vi "Magnetic Sweep 1.9.vi"() -> ()   [LabVIEW 2011]
panel:
  out "Current time":timestamp format="%<%I:%M:%S %p\n%x>T"
  out "error out":errorcluster
  in  "error in (no error) 2":errorcluster
  out "x .and. y?":bool
  in  "Initial Temperature":dbl
  out "Heater":bool
  out "Persistent switch ready":bool
  out "error out 6":errorcluster
  in  "Temperature\nlower limite":dbl
  out "Ramping rate command":string
  out "Target field command":string
  out "String":string="Persistent switch is not on"
  in  "Set parameter":bool
  out "status":string
  out "PID command":string
  out "setpoint command":string
  out "setpoint":dbl
  in  "stop":bool
  out "error out 3":errorcluster
  out "error out 2":errorcluster
  in  "Contour plot (ramp down)":path
  in  "Raw data (ramp down)":path
  out "Elapsed Time (s)":dbl format="%#_1g"
  out "Iteration":i32
  out "Zero field reached":bool
  out "Target field reached":bool
  in  "Temperature\nupper limite":dbl
  in  "Temperature\nramping step":dbl
  in  "Heater range":i16(ring) items=["High", "Medium", "Low"]
  in  "D gain":dbl
  in  "I gain":dbl
  in  "P gain":dbl
  in  "Contour plot (ramp up)":path
  in  "Timer":bool caption="Reset"
  in  "date format":enum16{"short", "long", "abbreviated"}(ring)
  in  "Save":bool
  in  "Raw data (ramp  up)":path
  out "Current Resistance":string
  out "Current Temperature":string
  out "Current Field":string
  out "Status":string
  in  "Field Sweep":bool
  in  "Magnetic field\nRamp rate":dbl
  in  "Traget Field":dbl
  out "Init Response":string
  in  "error in (no error)":errorcluster
  in  "IP Address":string
  in  "Update":bool
  in  "P Switch":bool
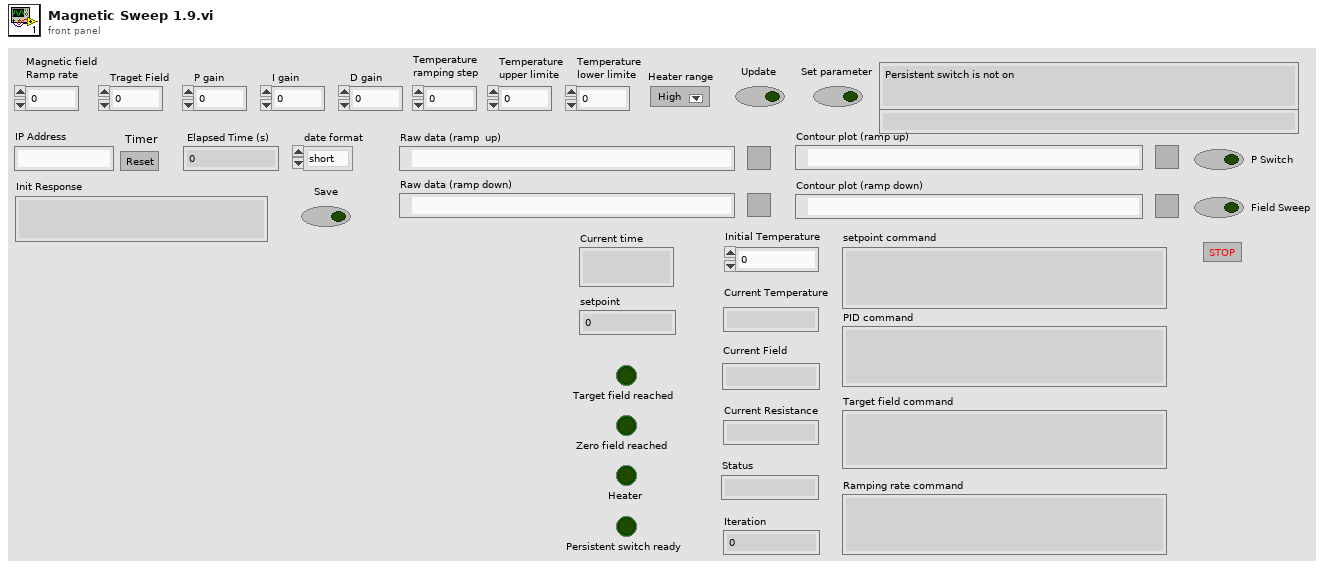
[diagram p1: front panel]
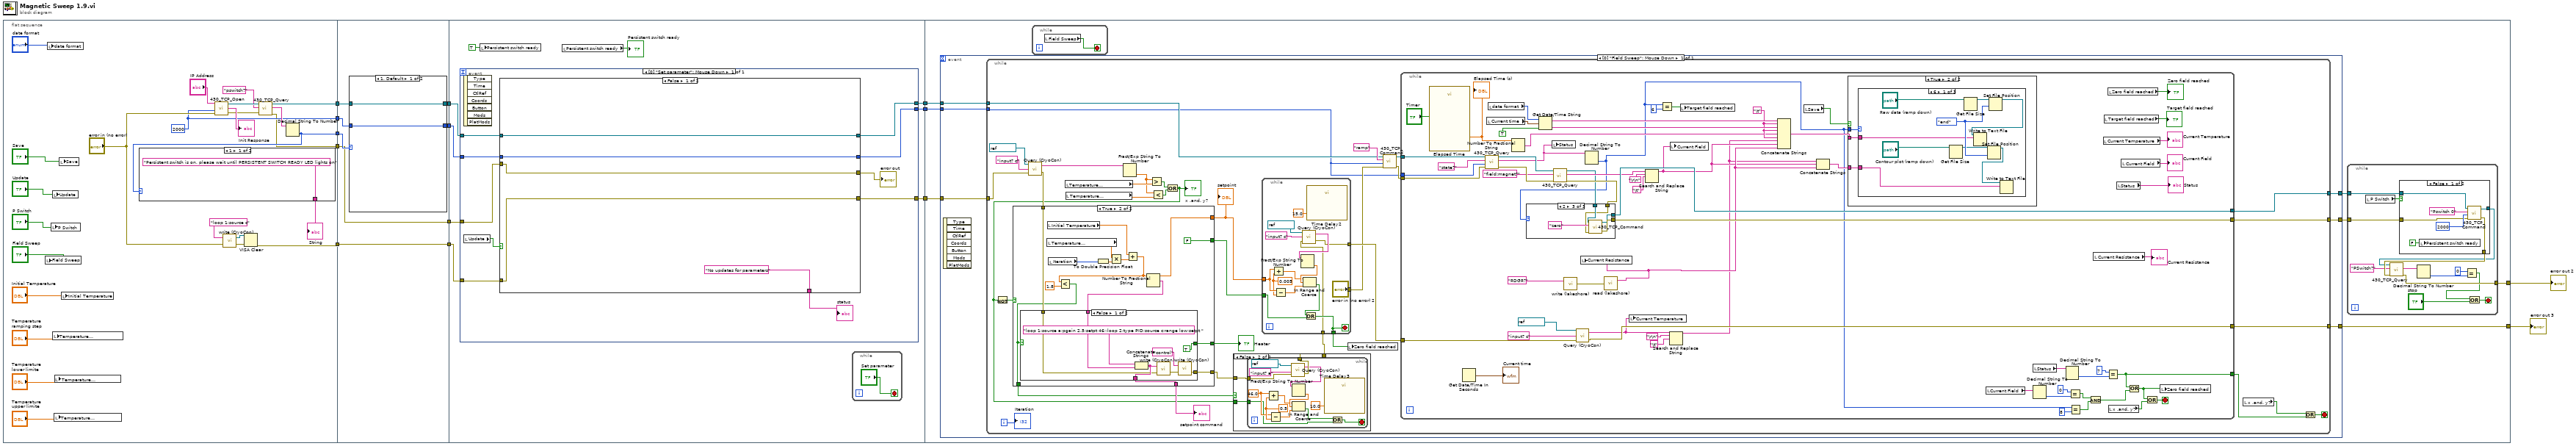
[diagram p0: block diagram]
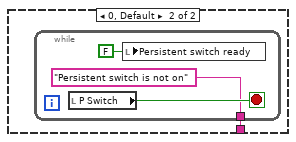
[diagram p2: hidden frame]
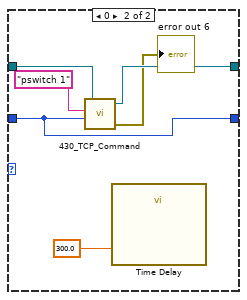
[diagram p3: hidden frame]
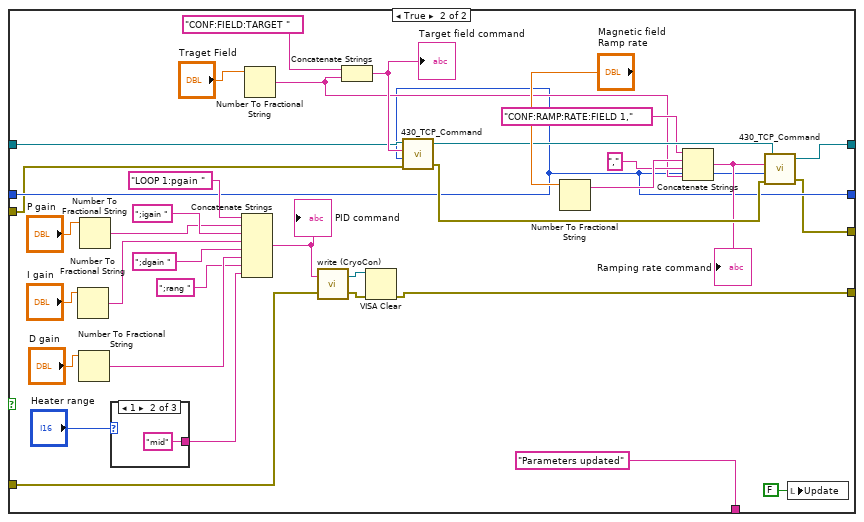
[diagram p4: hidden frame]
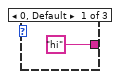
[diagram p5: hidden frame]
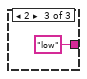
[diagram p6: hidden frame]
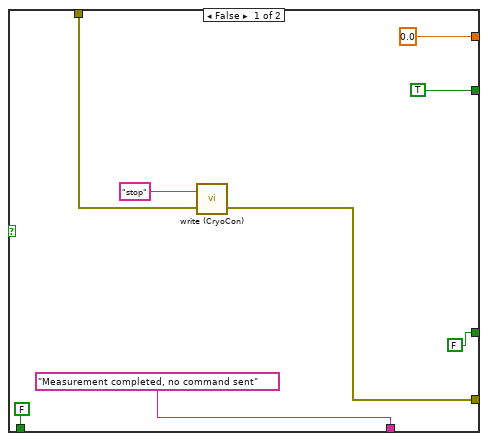
[diagram p9: hidden frame]
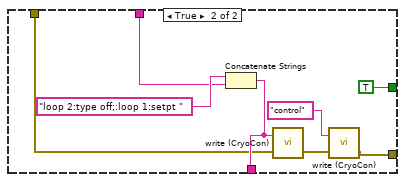
[diagram p10: hidden frame]
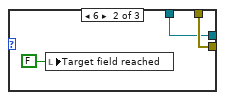
[diagram p12: hidden frame]
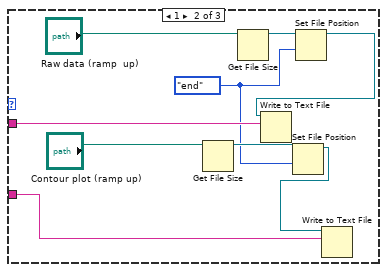
[diagram p14: hidden frame]
diagram:
  n1 = flat-sequence {
    tunnel: [w19] -> w11
    tunnel: [w21] -> w9
    tunnel: [w23] -> w7
    tunnel: [w18] -> w5
    tunnel: [w15] -> w1
    tunnel: w11 -> [w50]
    tunnel: [w48] -> w10
    tunnel: w9 -> [w49]
    tunnel: [w46] -> w8
    tunnel: w7 -> [w51]
    tunnel: [w51] -> w6
    tunnel: w5 -> [w47]
    tunnel: [w45] -> w2
    tunnel: w1 -> [w45]
    tunnel: w10 -> [w61]
    tunnel: w8 -> [w68]
    tunnel: w6 -> [w67]
    tunnel: [w66] -> w14
    tunnel: [w65] -> w13
    tunnel: [w64] -> w12
    tunnel: w2 -> [w60]
    tunnel: w14 -> [w129]
    tunnel: w13 -> [w126]
    tunnel: w12 -> [w125]
    tunnel: [w124] -> w4
    tunnel: [w123] -> w3
    frame #0 {
      w21 = 2000 ("Timeout")
      n2 = local write "Field Sweep"("Field Sweep") -> ()
      n3 = local write "date format"("date format") -> ()
      n4 = local write "P Switch"("P Switch") -> ()
      n5 = local write "Update"("Update") -> ()
      n6 = local write "Temperature\nramping step"("Temperature\nramping step") -> ()
      n7 = local write "Temperature\nupper limite"("Temperature\nupper limite") -> ()
      n8 = local write "Temperature\nlower limite"("Temperature\nlower limite") -> ()
      n9 = local write "Save"("Save") -> ()
      n10 = local write "Initial Temperature"("Initial Temperature") -> ()
      n11 = call "430_TCP_Open.vi"("IP Address"="IP Address", "timeout ms (2000)"=w21, "error in (no error)"="error in (no error)") -> ("connection ID"=w29:refnum<k5>, "Init Response"=→"Init Response":string, "error out"=w28:errorcluster)  [unwired: 3 in]
      n12 = call "write (CryoCon).vi"("error in (no error)"="error in (no error)", "write buffer"="loop 1:source c") -> ("error out"=w25:errorcluster, "VISA resource name out"=w24:refnum<visa-resource-name>)
      n13 = VISA Clear(VISA resource name=w24, error in (no error)=w25) -> (error out=w23:errorcluster)  [unwired: 1 out]
      n14 = call "430_TCP_Query.vi"("error in (no error)"=w28, "Command"="pswitch?", "connection ID"=w29) -> ("error out"=w15:errorcluster, "Response"=w26:string, "connection ID out"=w19:refnum<k5>)  [unwired: 4 in, 2 out]
      n15 = Decimal String To Number(string=w26) -> (number=w18:i32)  [unwired: 2 in, 1 out]
      n16 = case shown="1" w18 {
        tunnel: ["Persistent switch is on, please wait until PERSISTENT SWITCH READY LED lights on" w41] -> w22
        frame 1 {
        }
        frame 0, Default {
          n17 = while {
            tunnel: ["Persistent switch is not on"] -> w41
            stop <- w44 stop-if-true
            n18 = local read "P Switch"() -> (w44:bool)
            n19 = local write "Persistent switch ready"(FALSE ("Persistent switch ready")) -> ()
          }
        }
      }
      "String" <- w22
    }
    frame #1 {
      n20 = case shown="1, Default" w47 {
        tunnel: w50 -> [w53 w59]
        tunnel: w49 -> [w52 w54]
        tunnel: [w53 w58] -> w48
        tunnel: [w52 w54] -> w46
        frame 1, Default {
        }
        frame 0 {
          n21 = call "430_TCP_Command.vi"("Timeout"=w54, "Command"="pswitch 1", "connection ID"=w59) -> ("error out"=→"error out 6":errorcluster, "connection ID out"=w58:refnum<k5>)  [unwired: 1 in, 1 out]
          n22 = call "Time Delay"("Delay Time (s)"=300.0) -> ()  [unwired: 10 in, 1 out]
        }
      }
    }
    frame #2 {
      n23 = event shown="[0] \"Set parameter\": Mouse Down" {
        selector: _ -> [_]
        dyn-events: _ -> [_]
        timeout: _ -> [_]
        tunnel: w61 -> [w79]
        tunnel: w68 -> [w78]
        tunnel: w67 -> [w77]
        tunnel: [w76] -> w66
        tunnel: [w75] -> w65
        tunnel: [w74] -> w64
        tunnel: w60 -> [w71]
        event "Set parameter": Mouse Down {
          n24 = event-data() -> ()  [unwired: 1 in, 7 out]
          n25 = local read "Update"() -> (w72:bool)
          n26 = case shown="False" w72 {
            tunnel: w79 -> [w82 w117]
            tunnel: w78 -> [w83 w90]
            tunnel: w77 -> [w81 w96]
            tunnel: [w81 w86] -> w76
            tunnel: ["No updates for parameters" ("String") "Parameters updated" ("String")] -> w73
            tunnel: [w82 w91] -> w75
            tunnel: [w83 w90] -> w74
            tunnel: w71 -> [w80 w87]
            tunnel: [w80 w85] -> w70
            frame False {
            }
            frame True {
              n27 = Number To Fractional String(number="I gain") -> (F-format string=w100:string)  [unwired: 3 in]
              n28 = Number To Fractional String(number="D gain") -> (F-format string=w98:string)  [unwired: 3 in]
              n29 = Number To Fractional String(number="P gain") -> (F-format string=w101:string)  [unwired: 3 in]
              n30 = case shown="1" "Heater range" {
                tunnel: ["hi" "mid" "low"] -> w93
                frame 0, Default {
                }
                frame 1 {
                }
                frame 2 {
                }
              }
              n31 = Concatenate Strings("LOOP 1:pgain " ("write buffer"), w101, ";igain " ("string"), w100, ";dgain " ("string"), w98, ";rang " ("string"), w93) -> (w97:string)
              "PID command" <- w97
              n32 = Number To Fractional String(number="Traget Field") -> (F-format string=w107:string)  [unwired: 3 in]
              n33 = call "write (CryoCon).vi"("error in (no error)"=w96, "write buffer"=w97) -> ("error out"=w89:errorcluster, "VISA resource name out"=w88:refnum<visa-resource-name>)
              n34 = Concatenate Strings("CONF:FIELD:TARGET ", w107) -> (w118:string)
              "Target field command" <- w118
              n35 = VISA Clear(VISA resource name=w88, error in (no error)=w89) -> (error out=w86:errorcluster)  [unwired: 1 out]
              n36 = call "430_TCP_Command.vi"("error in (no error)"=w87, "Timeout"=w90, "Command"=w118, "connection ID"=w117) -> ("error out"=w116:errorcluster, "connection ID out"=w112:refnum<k5>)  [unwired: 1 out]
              n37 = Number To Fractional String(number="Magnetic field\nRamp rate") -> (F-format string=w110:string)  [unwired: 3 in]
              n38 = Concatenate Strings("CONF:RAMP:RATE:FIELD 1," ("string"), w110, "," ("string"), w107) -> (w113:string)
              "Ramping rate command" <- w113
              n39 = call "430_TCP_Command.vi"("error in (no error)"=w116, "Timeout"=w90, "Command"=w113, "connection ID"=w112) -> ("error out"=w85:errorcluster, "connection ID out"=w91:refnum<k5>)  [unwired: 1 out]
              n40 = local write "Update"(FALSE ("Update")) -> ()
            }
          }
          "status" <- w73
          "error out" <- w70
        }
      }
      n41 = local write "Persistent switch ready"(TRUE ("Persistent switch ready")) -> ()
      n42 = local read "Persistent switch ready"() -> (→"Persistent switch ready":bool)
      n43 = while {
        stop <- "Set parameter" stop-if-true
      }
    }
    frame #3 {
      n44 = event shown="[0] \"Field Sweep\": Mouse Down" {
        selector: _ -> [_]
        dyn-events: _ -> [_]
        timeout: _ -> [_]
        tunnel: w129 -> [w158]
        tunnel: [w157] -> w128
        tunnel: [w156] -> w127
        tunnel: w126 -> [w155]
        tunnel: w125 -> [w154]
        tunnel: [w153] -> w124
        event "Field Sweep": Mouse Down {
          n45 = event-data() -> ()  [unwired: 1 in, 7 out]
          n46 = while {
            tunnel: w158 -> [w175]
            tunnel: [w169] -> w157
            tunnel: [w188] -> w156
            tunnel: w155 -> [w187]
            tunnel: w154 -> [w159]
            tunnel: [w170] -> w153
            i -> [w191]
            stop <- w176 stop-if-true
            n47 = call "Query (CryoCon).vi"("error in (no error)"=w175, "write buffer"="input? c", "VISA resource name 2"=refnum<visa-resource-name> "COM3") -> ("error out"=w173:errorcluster, "read buffer"=w185:string)
            n48 = local read "Temperature\nupper limite"() -> (w189:dbl)
            n49 = local read "Temperature\nlower limite"() -> (w182:dbl)
            n50 = Fract/Exp String To Number(string=w185) -> (number=w183:dbl)  [unwired: 3 in, 1 out]
            n51 = Greater?(x=w183, y=w189) -> (0:w180:bool)
            n52 = Less?(x=w183, y=w182) -> (x < y?=w181:bool)
            n53 = Or(x=w180, y=w181) -> (x .or. y?=w160:bool)
            "x .and. y?" <- w160
            n54 = Not(x=w160) -> (.not. x?=w172:bool)
            n55 = case shown="True" w172 {
              tunnel: [w227 w242] -> w162
              tunnel: [0.0 w240] -> w192
              tunnel: ["Measurement completed, no command sent" w243] -> w171
              tunnel: [TRUE FALSE] -> w179
              tunnel: w173 -> [w229 w236]
              tunnel: [FALSE ("Heater") w235] -> w164
              tunnel: [FALSE w234] -> w163
              frame False {
                n56 = call "write (CryoCon).vi"("error in (no error)"=w229, "write buffer"="stop") -> ("error out"=w227:errorcluster)  [unwired: 1 out]
              }
              frame True {
                n57 = local read "Temperature\nramping step"() -> (w245:dbl)
                n58 = local read "Initial Temperature"() -> (w238:dbl)
                n59 = local read "Iteration"() -> (w237:i32)
                n60 = To Double Precision Float(number=w237) -> (double precision float=w244:dbl)
                n61 = Multiply(x=w245, y=w244) -> (x*y=w246:dbl)
                n62 = Add(x=w238, y=w246) -> (x+y=w240:dbl)
                n63 = Less?(x=w240, y=1.8) -> (x < y?=w234:bool)
                n64 = Number To Fractional String(number=w240) -> (F-format string=w247:string)  [unwired: 3 in]
                n65 = case shown="False" w234 {
                  tunnel: w247 -> [w254 w262]
                  tunnel: [w251 w261] -> w243
                  tunnel: [w253 w260] -> w242
                  tunnel: w236 -> [w248 w257]
                  tunnel: [TRUE ("Heater") TRUE ("Heater")] -> w235
                  frame False {
                    n66 = Concatenate Strings("loop 1:source a;pgain 2.5;setpt 46;:loop 2:type PID;source c;range low;setpt " ("write buffer"), w254) -> (w251:string)
                    n67 = call "write (CryoCon).vi"("error in (no error)"=w248, "write buffer"=w251) -> ("error out"=w250:errorcluster)  [unwired: 1 out]
                    n68 = call "write (CryoCon).vi"("error in (no error)"=w250, "write buffer"="control") -> ("error out"=w253:errorcluster)  [unwired: 1 out]
                  }
                  frame True {
                    n69 = Concatenate Strings("loop 2:type off;:loop 1:setpt " ("write buffer"), w262) -> (w261:string)
                    n70 = call "write (CryoCon).vi"("error in (no error)"=w257, "write buffer"=w261) -> ("error out"=w259:errorcluster)  [unwired: 1 out]
                    n71 = call "write (CryoCon).vi"("error in (no error)"=w259, "write buffer"="control") -> ("error out"=w260:errorcluster)  [unwired: 1 out]
                  }
                }
              }
            }
            "setpoint" <- w192
            "setpoint command" <- w171
            "Heater" <- w164
            n72 = case shown="False" w163 {
              tunnel: w162 -> [w193 w196]
              tunnel: [w193 w195] -> w161
              tunnel: w160 -> [_ w194]
              frame True {
              }
              frame False {
                n73 = while {
                  tunnel: w196 -> [w207]
                  tunnel: [w206] -> w195
                  tunnel: w194 -> [w198]
                  stop <- w197 stop-if-true
                  w200 = 46.0 ("x")
                  w201 = 0.5 ("y")
                  n74 = Add(x=w200, y=w201) -> (x+y=w203:dbl)
                  n75 = Subtract(x=w200, y=w201) -> (x-y=w202:dbl)
                  n76 = call "Query (CryoCon).vi"("error in (no error)"=w207, "write buffer"="input? a", "VISA resource name 2"=refnum<visa-resource-name> "COM3") -> ("error out"=w206:errorcluster, "read buffer"=w205:string)
                  n77 = Fract/Exp String To Number(string=w205) -> (number=w204:dbl)  [unwired: 3 in, 1 out]
                  n78 = In Range and Coerce(upper limit=w203, x=w204, lower limit=w202) -> (In Range?=w199:bool)  [unwired: 1 out]
                  n79 = call "Time Delay3"("Delay Time (s)"=10.0) -> ()  [unwired: 10 in, 1 out]
                  n80 = Or(x=w199, y=w198) -> (x .or. y?=w197:bool)
                }
              }
            }
            n81 = while {
              tunnel: w192 -> [w224]
              tunnel: w179 -> [w216]
              tunnel: [w214] -> w167
              tunnel: ["error in (no error) 2"] -> w166
              tunnel: [w212] -> w165
              tunnel: w161 -> [w211]
              stop <- w212 stop-if-true
              w221 = 0.005 ("y")
              n82 = Add(x=w224, y=w221) -> (x+y=w223:dbl)
              n83 = Subtract(x=w224, y=w221) -> (x-y=w222:dbl)
              n84 = call "Query (CryoCon).vi"("error in (no error)"=w211, "write buffer"="input? c", "VISA resource name 2"=refnum<visa-resource-name> "COM3") -> ("error out"=w214:errorcluster, "read buffer"=w218:string)
              n85 = Fract/Exp String To Number(string=w218) -> (number=w225:dbl)  [unwired: 3 in, 1 out]
              n86 = In Range and Coerce(upper limit=w223, x=w225, lower limit=w222) -> (In Range?=w215:bool)  [unwired: 1 out]
              n87 = Or(x=w215, y=w216) -> (x .or. y?=w212:bool)
              n88 = call "Time Delay2"("Delay Time (s)"=15.0) -> ()  [unwired: 10 in, 1 out]
            }
            n89 = local write "Zero field reached"(w165) -> ()
            n90 = call "430_TCP_Command.vi"("error in (no error)"=w166, "Timeout"=w159, "Command"="ramp", "connection ID"=w187) -> ("error out"=w168:errorcluster, "connection ID out"=w178:refnum<k5>)  [unwired: 1 out]
            n91 = while {
              tunnel: w178 -> [w316]
              tunnel: [w302] -> w170
              tunnel: [w304] -> w169
              tunnel: [w303] -> w188
              tunnel: [w276] -> w177
              tunnel: w168 -> [w288]
              tunnel: w167 -> [w287]
              tunnel: w159 -> [w283]
              stop <- w285 stop-if-true
              w318 = "\t"
              n92 = call "Elapsed Time"("Reset"="Timer") -> ("Elapsed Time (s)"=w312:dbl)  [unwired: 11 in, 7 out]
              "Elapsed Time (s)" <- w312
              n93 = Get Date/Time In Seconds() -> (seconds since 1Jan1904=→"Current time":timestamp)
              n94 = call "430_TCP_Query.vi"("error in (no error)"=w288, "Timeout"=w283, "Command"="state?", "connection ID"=w316) -> ("error out"=w282:errorcluster, "Response"=w267:string, "connection ID out"=w280:refnum<k5>)  [unwired: 3 in, 2 out]
              n95 = local read "Current time"() -> (w264:timestamp)
              n96 = local read "date format"() -> (w313:enum16{"short", "long", "abbreviated"})
              n97 = Number To Fractional String(number=w312) -> (F-format string=w314:string)  [unwired: 3 in]
              n98 = Get Date/Time String(date format (0)=w313, seconds (now)=w264, want seconds? (F)=TRUE) -> (date string=w320:string, time string=w319:string)
              n99 = local write "Status"(w267) -> ()
              n100 = call "430_TCP_Query.vi"("error in (no error)"=w282, "Command"="field:magnet?", "connection ID"=w280) -> ("error out"=w281:errorcluster, "Response"=w278:string, "connection ID out"=w277:refnum<k5>)  [unwired: 4 in, 2 out]
              n101 = call "write (lakeshore).vi"("write buffer"="RDGR?") -> ("error out"=w325:errorcluster)  [unwired: 1 in]
              n102 = call "Query (CryoCon).vi"("error in (no error)"=w287, "write buffer"="input? c", "VISA resource name 2"=refnum<visa-resource-name> "COM3") -> ("error out"=w302:errorcluster, "read buffer"=w299:string)
              n103 = Decimal String To Number(string=w267) -> (number=w266:i32)  [unwired: 2 in, 1 out]
              n104 = case shown="2" w266 {
                tunnel: [w328 w330 w335] -> w303
                tunnel: [w327 w329 w334] -> w304
                tunnel: w281 -> [w328 w330 w332]
                tunnel: w277 -> [w327 w329 w333]
                frame 0, Default {
                }
                frame 6 {
                  n105 = local write "Target field reached"(FALSE ("Target field reached")) -> ()
                }
                frame 2 {
                  n106 = call "430_TCP_Command.vi"("error in (no error)"=w332, "Command"="zero", "connection ID"=w333) -> ("error out"=w335:errorcluster, "connection ID out"=w334:refnum<k5>)  [unwired: 1 in, 1 out]
                }
              }
              n107 = call "read (lakeshore).vi"("error in (no error)"=w325) -> ("read buffer"=w294:string)  [unwired: 1 out]
              n108 = local write "Current Resistance"(w294) -> ()
              n109 = local write "Current Temperature"(w299) -> ()
              n110 = Search and Replace String(input string=w278, search string="\r\n", replace string="\t") -> (result string=w293:string)  [unwired: 5 in, 3 out]
              n111 = Equal?(x=w266, y=6) -> (x = y?=w315:bool)
              n112 = Search and Replace String(input string=w299, search string="\r\n", replace string="\t") -> (result string=w292:string)  [unwired: 5 in, 3 out]
              n113 = local write "Current Field"(w293) -> ()
              n114 = local write "Target field reached"(w315) -> ()
              n115 = Concatenate Strings(w320, w318, w319, w318, w314, w318, w292, w293, w294) -> (w323:string)
              n116 = local read "Save"() -> (w311:bool)
              n117 = Concatenate Strings(w292, w293, w294) -> (w317:string)
              n118 = case shown="True" w311 {
                tunnel: w323 -> [_ w339]
                tunnel: w317 -> [_ w338]
                tunnel: w266 -> [_ w337]
                frame False {
                }
                frame True {
                  n119 = case shown="6" w337 {
                    tunnel: w339 -> [w341 w357 _]
                    tunnel: w338 -> [w340 w351 _]
                    frame 6 {
                      w347 = enum16{"start", "end", "current"}."end" ("from (0:start)")
                      n120 = Get File Size(file="Contour plot (ramp down)") -> (refnum out=w346:refnum<file>)  [unwired: 1 in, 2 out]
                      n121 = Get File Size(file="Raw data (ramp down)") -> (refnum out=w343:refnum<file>)  [unwired: 1 in, 2 out]
                      n122 = Set File Position(refnum=w346, from (0:start)=w347) -> (refnum out=w348:refnum<file>)  [unwired: 2 in, 1 out]
                      n123 = Set File Position(refnum=w343, from (0:start)=w347) -> (refnum out=w344:refnum<file>)  [unwired: 2 in, 1 out]
                      n124 = Write to Text File(file (use dialog)=w344, text=w341) -> ()  [unwired: 2 in, 3 out]
                      n125 = Write to Text File(file (use dialog)=w348, text=w340) -> ()  [unwired: 2 in, 3 out]
                    }
                    frame 1 {
                      w350 = enum16{"start", "end", "current"}."end" ("from (0:start)")
                      n126 = Get File Size(file="Contour plot (ramp up)") -> (refnum out=w352:refnum<file>)  [unwired: 1 in, 2 out]
                      n127 = Get File Size(file="Raw data (ramp  up)") -> (refnum out=w355:refnum<file>)  [unwired: 1 in, 2 out]
                      n128 = Set File Position(refnum=w352, from (0:start)=w350) -> (refnum out=w349:refnum<file>)  [unwired: 2 in, 1 out]
                      n129 = Set File Position(refnum=w355, from (0:start)=w350) -> (refnum out=w354:refnum<file>)  [unwired: 2 in, 1 out]
                      n130 = Write to Text File(file (use dialog)=w354, text=w357) -> ()  [unwired: 2 in, 3 out]
                      n131 = Write to Text File(file (use dialog)=w349, text=w351) -> ()  [unwired: 2 in, 3 out]
                    }
                    frame Default {
                    }
                  }
                }
              }
              n132 = local read "Current Field"() -> (w272:string)
              n133 = local read "Status"() -> (w270:string)
              n134 = Decimal String To Number(string=w272) -> (number=w273:i32)  [unwired: 2 in, 1 out]
              n135 = Decimal String To Number(string=w270) -> (number=w269:i32)  [unwired: 2 in, 1 out]
              n136 = Equal?(x=0, y=w273) -> (x = y?=w290:bool)
              n137 = Equal?(x=w266, y=8) -> (x = y?=w291:bool)
              n138 = And(x=w290, y=w291) -> (x .and. y?=w289:bool)
              n139 = local read "Current Resistance"() -> (→"Current Resistance":string)
              n140 = local read "Current Temperature"() -> (→"Current Temperature":string)
              n141 = local read "Target field reached"() -> (→"Target field reached":bool)
              n142 = Equal?(x=7, y=w269) -> (x = y?=w276:bool)
              n143 = local read "Zero field reached"() -> (→"Zero field reached":bool)
              n144 = local read "x .and. y?"() -> (w284:bool)
              n145 = local read "Status"() -> (→"Status":string)
              n146 = local read "Current Field"() -> (→"Current Field":string)
              n147 = Or(x=w276, y=w289) -> (x .or. y?=w286:bool)
              n148 = Or(x=w286, y=w284) -> (x .or. y?=w285:bool)
              n149 = local write "Zero field reached"(w286) -> ()
            }
            n150 = local read "x .and. y?"() -> (w174:bool)
            n151 = Or(x=w174, y=w177) -> (x .or. y?=w176:bool)
            "Iteration" <- w191
          }
        }
      }
      n152 = while {
        stop <- w130 stop-if-true
        n153 = local read "Field Sweep"() -> (w130:bool)
      }
      n154 = while {
        tunnel: w128 -> [w143]
        tunnel: w127 -> [w141]
        tunnel: [w136] -> w123
        stop <- w131 stop-if-true
        n155 = local read "P Switch"() -> (w142:bool)
        n156 = case shown="False" w142 {
          tunnel: w143 -> [w149 w152]
          tunnel: w141 -> [w147 w151]
          tunnel: [w145 w151] -> w139
          tunnel: [w144 w152] -> w138
          frame False {
            n157 = local write "Persistent switch ready"(FALSE ("Persistent switch ready")) -> ()
            n158 = call "430_TCP_Command.vi"("error in (no error)"=w147, "Timeout"=2000, "Command"="Pswitch 0", "connection ID"=w149) -> ("error out"=w145:errorcluster, "connection ID out"=w144:refnum<k5>)  [unwired: 1 out]
          }
          frame True {
          }
        }
        n159 = call "430_TCP_Query.vi"("error in (no error)"=w139, "Command"="PSwitch?", "connection ID"=w138) -> ("error out"=w136:errorcluster, "Response"=w135:string)  [unwired: 4 in, 3 out]
        n160 = Decimal String To Number(string=w135) -> (number=w134:i32)  [unwired: 2 in, 1 out]
        n161 = Equal?(x=0, y=w134) -> (x = y?=w132:bool)
        n162 = Or(x=w132, y="stop") -> (x .or. y?=w131:bool)
      }
    }
  }
  "error out 2" <- w3
  "error out 3" <- w4
